vi "DCC_get_overload_state.vi"(8 "Error In":errorcluster, 10 "Module No":i16, 11 "DLL Path":path) -> (0 "Error Out":errorcluster, 2 "Module No":i16, 3 "DLL Path":path, 4 "State":i16, 5 "Overload Status":cluster{"Connector 2":bool, "Connector 1":bool})   [LabVIEW 2017]
doc: "The procedure is used to check whether an overload occurred on the DCC module ‘mod_no’.\n\nBit 0 of the ‘state’ variable is set when Connector 1 Overload is present, otherwise it is 0.\nBit 1 of the ‘state’ variable is set when Connector 3 Overload is present, otherwise it is 0.\n\nAugust 2018\nFrank Quadt & Stefan Smietana\ninfo@becker-hickl.com"
panel:
  # "(c) 2021 Becker & Hickl GmbH\n     All Rights Reserved."
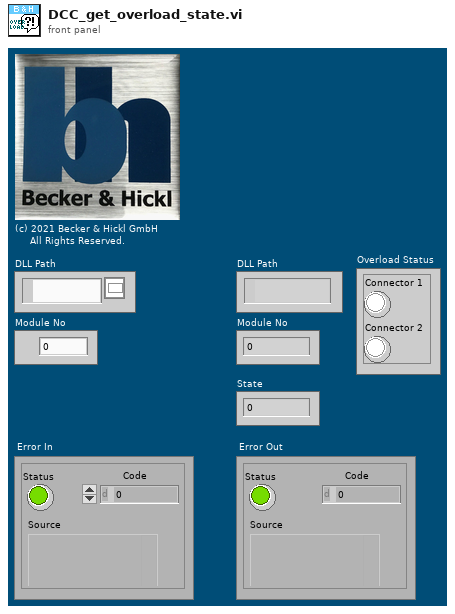
[diagram p1: front panel]
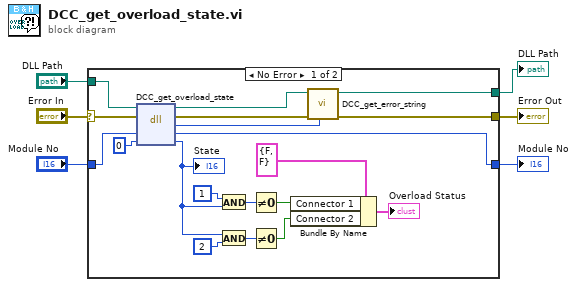
[diagram p0: block diagram]
diagram:
  n1 = case shown="No Error" "Error In" {
    selector: "Error In" -> [w25 w27]
    tunnel: [w18 w27] -> w5
    tunnel: [w20 w26] -> w4
    tunnel: "DLL Path" -> [w23 w26]
    tunnel: [w22 w28] -> w2
    tunnel: "Module No" -> [w21 w28]
    frame No Error {
      n2 = dll-call lib="C:/Program Files/BH/DCC/DLL/dcc32.dll" fn="DCC_get_overload_state"(path in=w23, error in=w25, "ModuleNo"=w21, "State"=i16 0) -> (path out=w24:path, error out=w19:errorcluster, "return type"=w17:i16, "ModuleNo"=w22:i16, "State"=w13:i16)  [unwired: 1 in]
      "State" <- w13
      n3 = And(x=i16 1, y=w13) -> (x .and. y?=w11:i16)
      n4 = And(x=w13, y=i16 2) -> (x .and. y?=w10:i16)
      n5 = Not Equal To 0?(x=w11) -> (x != 0?=w9:bool)
      n6 = Not Equal To 0?(x=w10) -> (x != 0?=w8:bool)
      n7 = Bundle By Name(cluster=cluster{"Connector 2":bool, "Connector 1":bool} {"Connector 2"=FALSE, "Connector 1"=FALSE} ("Overload Status 2"), "Connector 1"=w9, "Connector 2"=w8) -> (→"Overload Status":cluster{"Connector 2":bool, "Connector 1":bool})
      n8 = call "DCC_get_error_string.vi"("Error ID"=w17, "Error In"=w19, "DLL Path"=w24) -> ("Error Out"=w18:errorcluster, "DLL Path"=w20:path)  [unwired: 6 in, 1 out]
    }
    frame Error {
    }
  }
  "Error Out" <- w5
  "DLL Path" <- w4
  "Module No" <- w2
